vi "Set Exposure.vi"(4 "DesiredHist":i32=120, 6 "UnderThr":bool=TRUE, 7 "ExpGain":i32=-100, 8 "Image":T1, 9 "Exposure":u32=62000, 10 "AutoExposure":bool=TRUE, 11 "Session Out":T2) -> (1 "ActualExposure":u32, 2 "HistMax":i32)   [LabVIEW 2015]
uses:
  <vilib>/userdefined/High Color/IMAQdx.ctl
  <vilib>/vision/Image Controls.llb/IMAQ Image.ctl
  Belkin Globals.vi
  <resource>/objmgr/imaqdx.rc
  <vilib>/vision/NI_Vision_Development_Module.lvlib
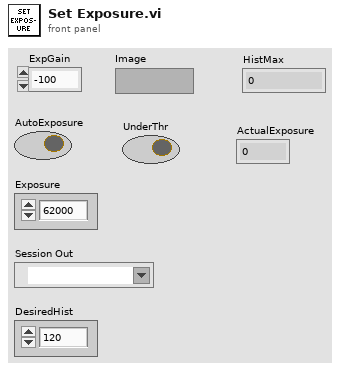
[diagram p1: front panel]
types:
  T1 = typedef "IMAQ Image.ctl" = refnum<image>
  T2 = typedef "IMAQdx.ctl" = refnum<k21>
  T3 = cluster{"histogram":u32[], "Minimal Value":sgl, "Maximal Value":sgl, "Starting Value":sgl, "Interval Width":sgl, "Mean Value":sgl, "Standard  Variation":sgl, "Area (pixels)":i32}
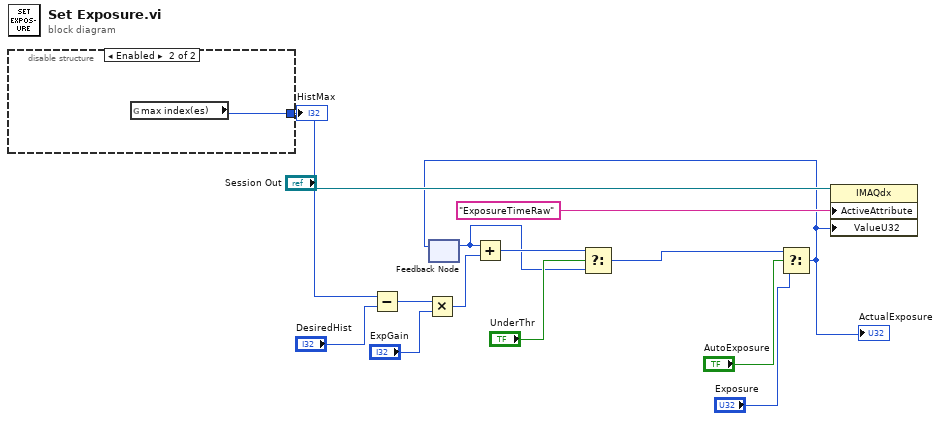
[diagram p0: block diagram]
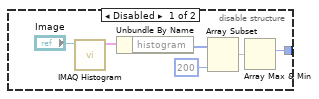
[diagram p2: hidden frame]
diagram:
  n1 = disable-structure shown="Enabled" {
    disable-tunnel: [w15 w21] -> w6
    frame Disabled {
      n2 = call "IMAQ Histogram"("Image"="Image") -> ("Histogram Report"=w20:T3)  [unwired: 9 in, 1 out]
      n3 = Unbundle By Name(w20) -> ("histogram"=w19:u32[])
      n4 = Array Subset(array=w19, length=200) -> (w17:u32[])  [unwired: 1 in]
      n5 = Array Max & Min(array=w17) -> (max index (indices)=w15:i32)  [unwired: 3 out]
    }
    frame Enabled {
      n6 = global read "Belkin Globals.vi" "max index(es)"() -> (w21:i32)
    }
  }
  "HistMax" <- w6
  n7 = Subtract(x=w6, y="DesiredHist") -> (x-y=w10:i32)
  n8 = Multiply(x=w10, y="ExpGain") -> (x*y=w12:i32)
  n9 = feedback #1() -> (w1:u32)  [unwired: 1 in]
  n10 = Add(x=w1, y=w12) -> (x+y=w3:u32)
  n11 = Select(t=w3, s="UnderThr", f=w1) -> (s? t:f=w2:u32)
  n12 = Select(t=w2, s="AutoExposure", f="Exposure") -> (s? t:f=w4:u32)
  "ActualExposure" <- w4
  n13 = feedback-in #1(w4) -> ()
  n14 = property class="IMAQdx"(reference="Session Out", "ActiveAttribute"="ExposureTimeRaw", "ValueU32"=w4) -> ()  [unwired: 1 in, 2 out]
